vi "Interpolate Y (multiple).vi"(8 "error in (no error)":errorcluster, 10 "x (0)":dbl, 11 "XY-data":cluster{"X-array":dbl[], "Y-array":dbl[]}[](array[cluster])) -> (0 "error out":errorcluster, 2 "y":dbl[](array[numeric]), 3 "XY-data out":cluster{"X-array":dbl[], "Y-array":dbl[]}[](array[cluster]) {"Y-array" format="%.2p"; "X-array" format="%.2p"})   [LabVIEW 2016, in "xy_utilities.lvlib"]
doc: "Given a fractional <b>x</b> value, interpolate a factional <b>y</b> value.\n\nWire data to the data input to determine the polymorphic instance to use or manually select the instance."
uses:
  xy_utilities.lvlib
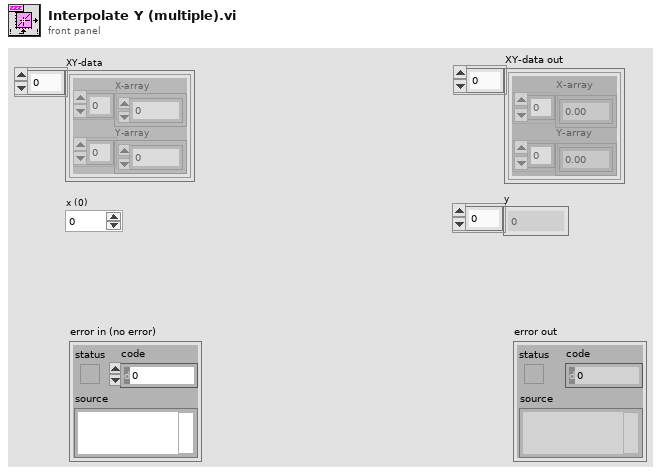
[diagram p1: front panel]
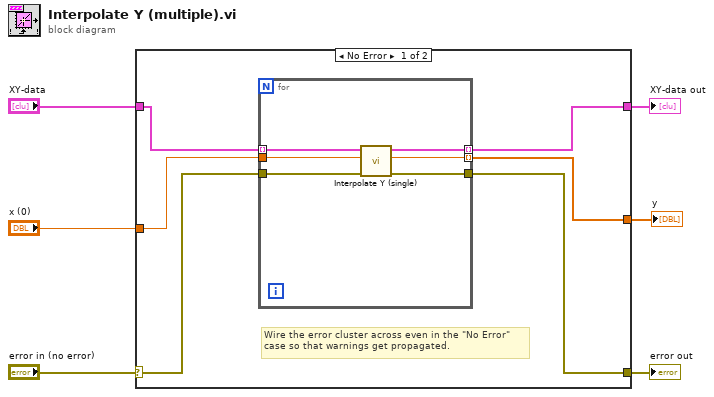
[diagram p0: block diagram]
diagram:
  n1 = case shown="No Error" "error in (no error)" {
    selector: "error in (no error)" -> [w12 w20]
    tunnel: [w8 w20] -> w5
    tunnel: "XY-data" -> [w7 w19]
    tunnel: [w10 w19] -> w3
    tunnel: "x (0)" -> [w11 _]
    tunnel: [w9 _] -> w1
    frame No Error {
      # "Wire the error cluster across even in the \"No Error\"\ncase so that warnings get propagated."
      n2 = for {
        tunnel: w12 -> [w18]
        tunnel: w11 -> [w17]
        tunnel: w7 -> [w16] mode=indexing
        tunnel: [w15] -> w10 mode=indexing
        tunnel: [w14] -> w9 mode=indexing
        tunnel: [w13] -> w8
        n3 = call "Interpolate Y (single).vi"("error in (no error)"=w18, "x (0)"=w17, "XY-data"=w16) -> ("error out"=w13:errorcluster, "y"=w14:dbl, "XY-data out"=w15:cluster{"X-array":dbl[], "Y-array":dbl[]})  [unwired: 6 in]
      }
    }
    frame Error {
    }
  }
  "error out" <- w5
  "XY-data out" <- w3
  "y" <- w1
